vi "calc_C_flocculated.vi"(3 "RowData":T1) -> (0 "RowData 2":T1)   [LabVIEW 2019]
uses:
  RowData_Type.ctl
  Global Plantita Parameters.vi
panel:
  # "Inputs"
  # "Outputs"
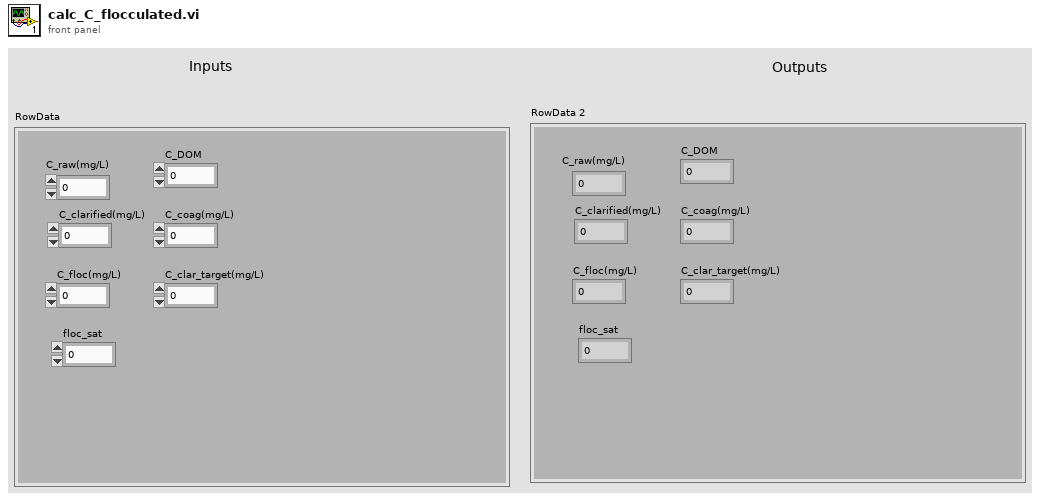
[diagram p1: front panel]
types:
  T1 = typedef "RowData_Type.ctl" = cluster{"C_raw(mg/L)":dbl, "C_clarified(mg/L)":dbl, "C_floc(mg/L)":dbl, "floc_sat":dbl, "C_DOM":dbl, "C_coag(mg/L)":dbl, "C_clar_target(mg/L)":dbl}
  T2 = cluster{"height_ff (m)":dbl, "C_coag_stock (g/L)":dbl, "flocculation_time(min)":dbl, "clarification_time(min)":dbl, "data_interval (min)":dbl, "kpf":dbl, "kc":dbl, "q":dbl}
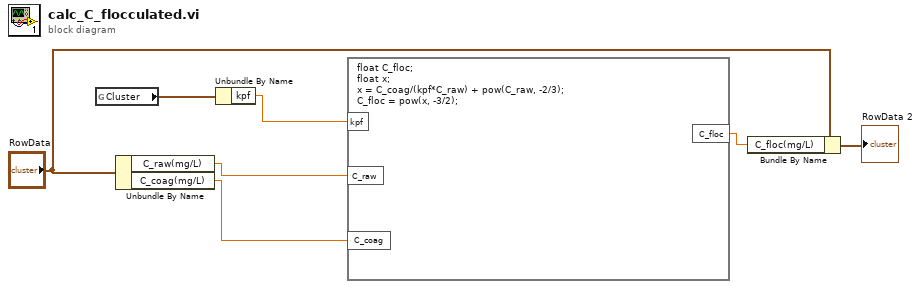
[diagram p0: block diagram]
diagram:
  n1 = global read "Global Plantita Parameters.vi" "Cluster"() -> (w2:T2)
  n2 = Unbundle By Name("RowData") -> ("C_raw(mg/L)"=w3:dbl, "C_coag(mg/L)"=w4:dbl)
  n3 = Unbundle By Name(w2) -> ("kpf"=w1:dbl)
  n4 = formula code="float C_floc;\nfloat x;\nx = C_coag/(kpf*C_raw) + pow(C_raw, -2/3);\nC_floc = pow(x, -3/2);"("kpf"=w1, "C_raw"=w3, "C_coag"=w4) -> ("C_floc"=w6:dbl)
  n5 = Bundle By Name(cluster="RowData", "C_floc(mg/L)"=w6) -> (→"RowData 2":T1)
